vi "Stop Core.vi"(10 "final error code":i32, 11 "Grid Animation in":refnum<class "Grid Animation.lvclass">) -> (3 "Grid Animation out":refnum<class "Grid Animation.lvclass">)   [LabVIEW 2021, in "Grid Animation.lvlib" / "Grid Animation.lvclass"]
doc: "<p>(<strong>Filename</strong>: <span class=\"dnl\">Actor Framework.lvlib:Actor.lvclass:Stop Core.vi</span>)</p>\n<p>Defines what the actor does before it stops. Use the <strong>final error code</strong> input to determine whether the actor shut down in response to an error.</p>\n<p>By default, this method passes the Stop message along to all <a href=\"nihelplauncher://docs/csh?context=lvcore_lvcomm_af_launch_nested_actor\">auto-stop nested actors</a>. A descendant class may override this method to define additional behavior, such as shutting down any processes the actor initiated in its override of the <a href=\"nihelplauncher://docs/csh?context=lvcore_lvcomm_af_actor_core\">Actor Core</a> method.</p>"
uses:
  Grid Animation.lvclass
  Grid Animation.lvclass/Grid Animation.ctl
  MC Screen/Grid Screen Messages/Set Grid Value Using Coordinates Msg/Set Grid Value Using Coordinates Msg.lvclass/Set Grid Value Using Coordinates Msg.ctl
  <vilib>/ActorFramework/Message Enqueuer/Message Enqueuer.lvclass/Message Enqueuer.ctl
  <vilib>/ActorFramework/Message Enqueuer/Enqueue.vi
  MC Screen/Grid Screen Messages/Set Grid Value Using Coordinates Msg/Set Grid Value Using Coordinates Msg.lvclass
  C:/Program Files/National Instruments/LabVIEW 2024/vi.lib/ActorFramework/Message/Message.lvclass
  <vilib>/ActorFramework/Message Priority Queue/Priority Enqueue.vi
  <vilib>/ActorFramework/Actor/Actor.lvclass
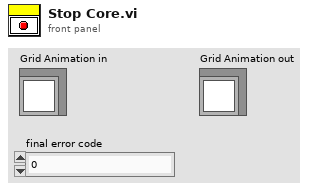
[diagram p1: front panel]
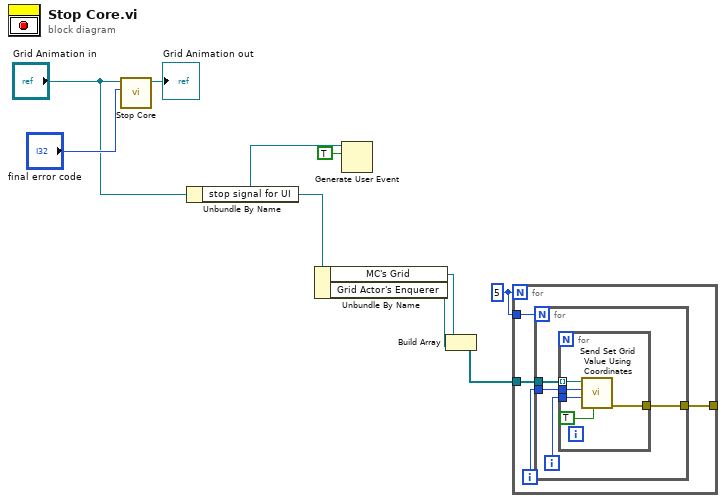
[diagram p0: block diagram]
diagram:
  w2 = 5
  n1 = call-parent "Stop Core.vi"("final error code"="final error code", "Actor in"="Grid Animation in") -> ("Actor out"=→"Grid Animation out":refnum<class "Grid Animation.lvclass">)  [unwired: 9 in]
  n2 = Unbundle By Name("Grid Animation in") -> ("stop signal for UI"=w6:refnum<user-event>)
  n3 = Unbundle By Name("Grid Animation in") -> ("MC's Grid"=w5:refnum<class "Message Enqueuer.lvclass">, "Grid Actor's Enquerer"=w4:refnum<class "Message Enqueuer.lvclass">)
  n4 = Generate User Event(user event=w6, event data cluster=TRUE ("event data")) -> ()  [unwired: 2 in, 2 out]
  n5 = Build Array(w5, w4) -> (w3:refnum<class "Message Enqueuer.lvclass">[])
  n6 = for {
    N: w2 -> [_]
    tunnel: w3 -> [w13]
    tunnel: w2 -> [w12]
    tunnel: [w10] -> _
    i -> [w11]
    n7 = for {
      N: w12 -> [_]
      tunnel: w13 -> [w17]
      tunnel: w11 -> [w16]
      tunnel: [w14] -> w10
      i -> [w15]
      n8 = for {
        tunnel: w17 -> [w22] mode=indexing
        tunnel: w16 -> [w21]
        tunnel: w15 -> [w20]
        tunnel: [w18] -> w14
        n9 = call "Send Set Grid Value Using Coordinates.vi"("Cell Value"=TRUE, "Row"=w20, "Column"=w21, "Message Enqueuer"=w22) -> ("error out"=w18:errorcluster)  [unwired: 6 in, 1 out]
      }
    }
  }
